vi "Construct.vi"(6 "Bulk Size (1)":i32=1, 7 "Use system decimal point (F)":bool, 8 "error in (no error)":errorcluster, 9 "Constants":cluster{"name":string, "value":dbl}[](array[cluster]), 10 "Expression":string, 11 "muExpr in":refnum<class "mupExpr.lvclass">) -> (0 "error out":errorcluster, 1 "error details":T1, 2 "Variable Names":string[](array[string]), 3 "mupExpr out":refnum<class "mupExpr.lvclass">)   [LabVIEW 2015, in "mupExpr.lvclass"]
doc: "Construct a new muExpr instance. Input an expression or a set of expressions.\nReturns the expression handle and the list of variables found in the expression.\n\nOptionally input a list of constant name-value pairs.\n\nSet \"Use system decimal point\" to true if you want to adapt to the system's decimal point. If the system's decimal point is a comma, the argument separator will be changed to a semi-colon. The default decimal point is a period. The default argument separator is a comma.\n\nSet Bulk Size sets the range for bulk mode evaluations. Default is 1 (single result)."
uses:
  mupExpr.lvclass
  mupExpr.lvclass/mupExpr.ctl
  mupLib/mupLibPath.vi
  mupLib/mupCheckError.vi
  <vilib>/Utility/error.llb/Error Cluster From Error Code.vi
  mupLib/mupLib.lvlib
panel:
  # "Construct a new muExpr instance. Input an expression or a set of expressions.\nReturns the expression handle and the list of variables found in the expression (for convenience)."
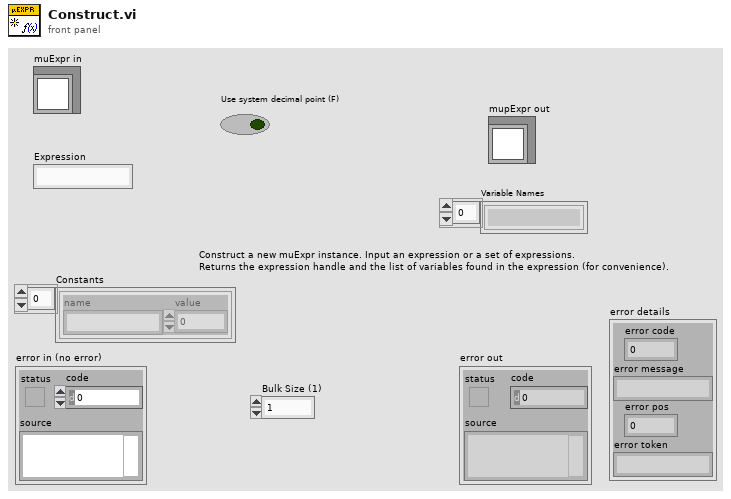
[diagram p1: front panel]
types:
  T1 = cluster{"error code":i32, "error message":string, "error pos":i32, "error token":string}
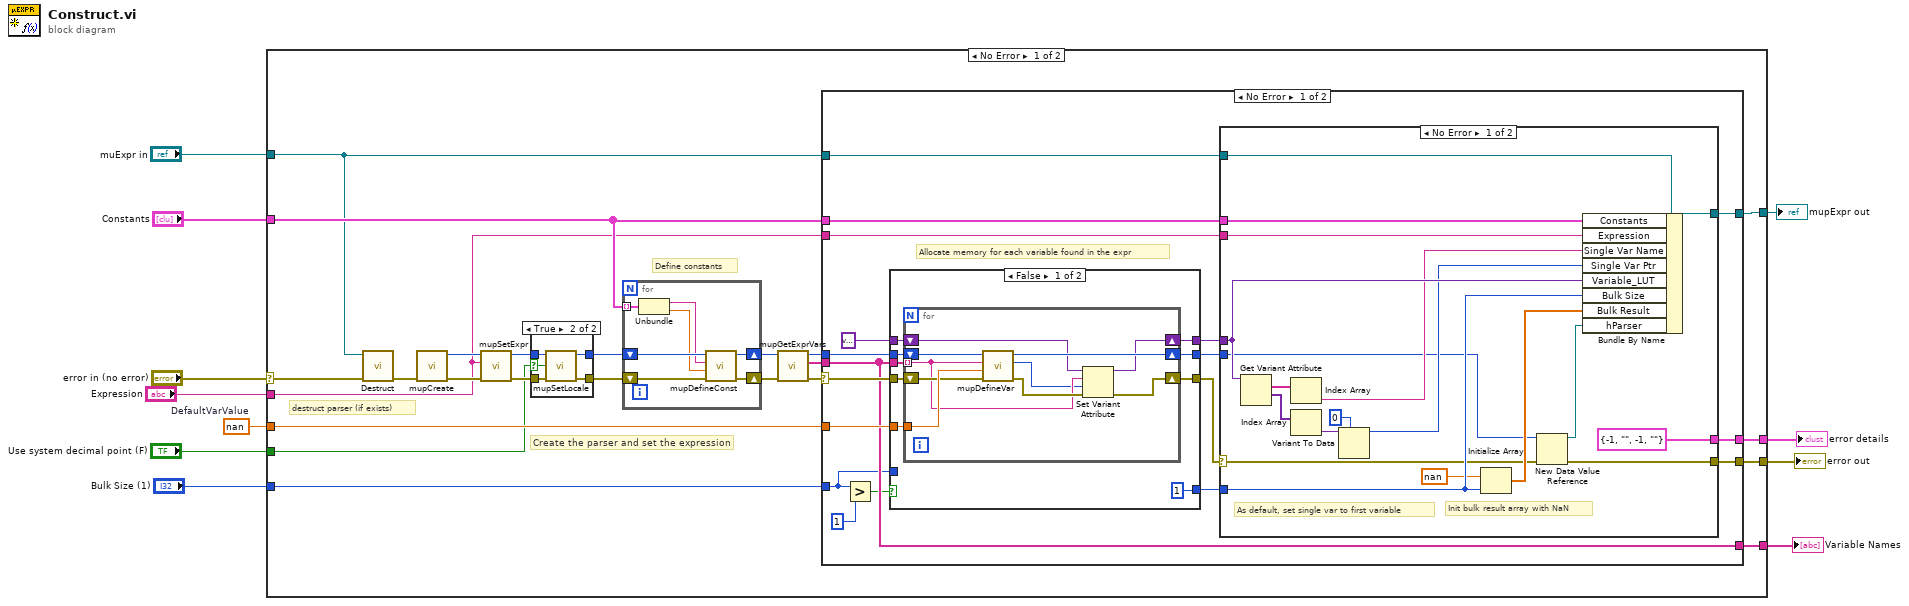
[diagram p0: block diagram]
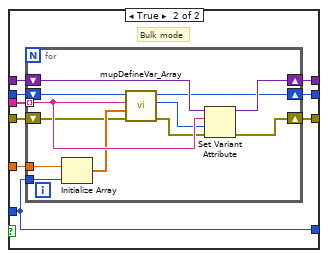
[diagram p3: hidden frame]
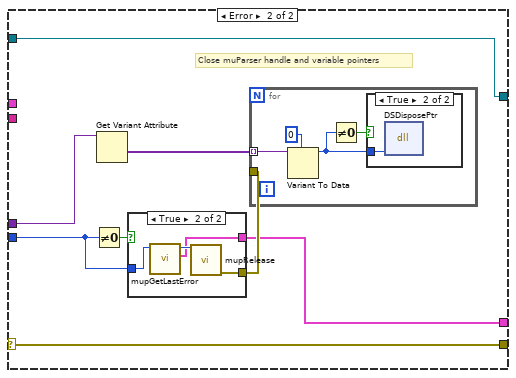
[diagram p4: hidden frame]
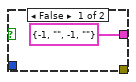
[diagram p5: hidden frame]
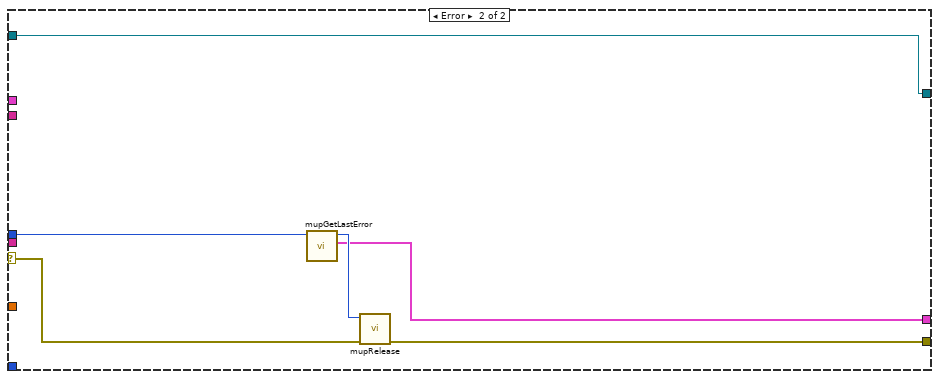
[diagram p7: hidden frame]
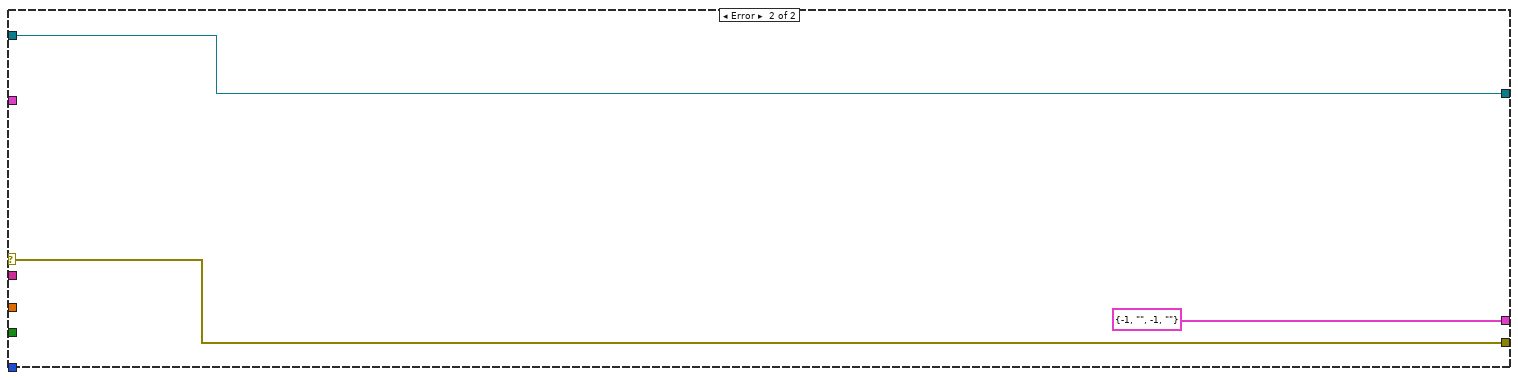
[diagram p8: hidden frame]
diagram:
  w8 = nan  # DefaultVarValue
  n1 = case shown="No Error" "error in (no error)" {
    selector: "error in (no error)" -> [w14 w152]
    tunnel: "Expression" -> [w12 _]
    tunnel: [w34 w150] -> w3
    tunnel: [w33 w152] -> w10
    tunnel: w8 -> [w32 _]
    tunnel: [w31 _] -> w7
    tunnel: "Use system decimal point (F)" -> [w19 _]
    tunnel: "Constants" -> [w17 _]
    tunnel: "Bulk Size (1)" -> [w18 _]
    tunnel: [w16 T1 {"error code"=-1, "error message"="", "error pos"=-1, "error token"=""} ("error details")] -> w2
    tunnel: "muExpr in" -> [w15 w150]
    frame No Error {
      # "destruct parser (if exists)"
      # "Define constants"
      # "Create the parser and set the expression"
      n2 = call-dynamic "Destruct.vi"("error in (no error)"=w14, "muExpr in"=w15) -> ("error out"=w13:errorcluster)  [unwired: 9 in]
      n3 = call "mupCreate.vi"("error in (no error)"=w13) -> ("error out"=w26:errorcluster, "hParser out"=w27:u64)  [unwired: 9 in]
      n4 = call "mupSetExpr.vi"("error in (no error)"=w26, "szExpr"=w12, "muPar in"=w27) -> ("error out"=w25:errorcluster, "muPar out"=w24:u64)  [unwired: 7 in]
      n5 = case shown="True" w19 {
        selector: w19 -> [_ w37]
        tunnel: w25 -> [w35 w41]
        tunnel: w24 -> [w36 w40]
        tunnel: [w36 w39] -> w23
        tunnel: [w35 w38] -> w21
        frame False {
        }
        frame True {
          n6 = call "mupSetLocale.vi"("error in (no error)"=w41, "Use system decimal point (T)"=w37, "hParser in"=w40) -> ("error out"=w38:errorcluster, "hParser out"=w39:u64)  [unwired: 7 in]
        }
      }
      n7 = for {
        shift-right: [w47] -> w22
        shift-left: w23 -> [w48]
        shift-right: [w45] -> w20
        shift-left: w21 -> [w46]
        tunnel: w17 -> [w44] mode=indexing
        n8 = Unbundle(w44) -> ("name"=w43:string, "value"=w42:dbl)
        n9 = call "mupDefineConst.vi"("error in (no error)"=w46, "Value"=w42, "constName"=w43, "hParser in"=w48) -> ("error out"=w45:errorcluster, "hParser out"=w47:u64)  [unwired: 6 in]
      }
      n10 = call "mupGetExprVars.vi"("error in (no error)"=w20, "hParser in"=w22) -> ("error out"=w29:errorcluster, "varNames"=w28:string[], "hParser out"=w30:u64)  [unwired: 5 in, 2 out]
      n11 = case shown="No Error" w29 {
        selector: w29 -> [w61 w146]
        tunnel: [w66 w144] -> w34
        tunnel: [w65 w149] -> w33
        tunnel: w32 -> [w62 _]
        tunnel: w30 -> [w63 w147]
        tunnel: [w57 _] -> w31
        tunnel: w28 -> [w57 _]
        tunnel: w18 -> [w54 _]
        tunnel: w17 -> [w53 _]
        tunnel: [w51 w145] -> w16
        tunnel: w15 -> [w50 w144]
        tunnel: w12 -> [w49 _]
        frame No Error {
          # "Allocate memory for each variable found in the expr"
          n12 = Greater?(x=w54, y=1) -> (0:w55:bool)
          n13 = case shown="False" w55 {
            tunnel: variant -> [w75 w94]
            tunnel: w63 -> [w74 w93]
            tunnel: w62 -> [w73 w92]
            tunnel: w61 -> [w72 w91]
            tunnel: [w71 w90] -> w60
            tunnel: [w70 w89] -> w59
            tunnel: [w69 w88] -> w58
            tunnel: w57 -> [w68 w87]
            tunnel: w54 -> [_ w86]
            tunnel: [1 ("Bulk Size (1)") w86] -> w52
            frame False {
              n14 = for {
                tunnel: w68 -> [w78] mode=indexing
                shift-right: [w79] -> w69
                shift-left: w75 -> [w80]
                shift-right: [w84] -> w70
                shift-left: w74 -> [w85]
                tunnel: w73 -> [w83]
                shift-right: [w76] -> w71
                shift-left: w72 -> [w82]
                n15 = call "mupDefineVar.vi"("error in (no error)"=w82, "initValue"=w83, "varName"=w78, "hParser in"=w85) -> ("error out"=w81:errorcluster, "varAddr"=w77:u64, "hParser out"=w84:u64)  [unwired: 5 in]
                n16 = Set Variant Attribute(Variant=w80, name=w78, value=w77, error in=w81) -> (Variant out=w79:variant, error out=w76:errorcluster)  [unwired: 1 out]
              }
            }
            frame True {
              # "Bulk mode"
              n17 = for {
                tunnel: w87 -> [w99] mode=indexing
                shift-right: [w105] -> w88
                shift-left: w94 -> [w106]
                shift-right: [w100] -> w89
                shift-left: w93 -> [w101]
                tunnel: w92 -> [w103]
                shift-right: [w104] -> w90
                shift-left: w91 -> [w97]
                tunnel: w86 -> [w102]
                n18 = Initialize Array(w103, w102) -> (w98:dbl[])
                n19 = call "mupDefineVar_Array.vi"("error in (no error)"=w97, "initValue"=w98, "varName"=w99, "hParser in"=w101) -> ("error out"=w96:errorcluster, "varAddr"=w95:u64, "hParser out"=w100:u64)  [unwired: 5 in]
                n20 = Set Variant Attribute(Variant=w106, name=w99, value=w95, error in=w96) -> (Variant out=w105:variant, error out=w104:errorcluster)  [unwired: 1 out]
              }
            }
          }
          n21 = case shown="No Error" w60 {
            selector: w60 -> [w107 w129]
            tunnel: [w113 w126] -> w66
            tunnel: w59 -> [w109 w132]
            tunnel: w58 -> [w125 w131]
            tunnel: [w110 w129] -> w65
            tunnel: w53 -> [w118 _]
            tunnel: w52 -> [w117 _]
            tunnel: [T1 {"error code"=-1, "error message"="", "error pos"=-1, "error token"=""} ("error details") w127] -> w51
            tunnel: w50 -> [w112 w126]
            tunnel: w49 -> [w108 _]
            frame No Error {
              # "As default, set single var to first variable"
              # "Init bulk result array with NaN"
              n22 = Get Variant Attribute(Variant=w125) -> (names=w124:string[], values=w123:variant[])  [unwired: 3 in, 2 out]
              n23 = Index Array(array=w124) -> (element=w120:string)  [unwired: 1 in]
              n24 = Index Array(array=w123) -> (element=w122:variant)  [unwired: 1 in]
              n25 = Variant To Data(type=u64 0, Variant=w122) -> (data=w119:u64)  [unwired: 1 in, 1 out]
              n26 = Initialize Array(nan ("element"), w117) -> (w115:dbl[])
              n27 = New Data Value Reference(data value=w109, error in=w107) -> (data value reference=w111:refnum<data-value>, error out=w110:errorcluster)
              n28 = Bundle By Name(cluster=w112, "Constants"=w118, "Expression"=w108, "Single Var Name"=w120, "Single Var Ptr"=w119, "Variable_LUT"=w125, "Bulk Size"=w117, "Bulk Result"=w115, "hParser"=w111) -> (w113:refnum<class "mupExpr.lvclass">)
            }
            frame Error {
              # "Close muParser handle and variable pointers"
              n29 = Not Equal To 0?(x=w132) -> (x != 0?=w133:bool)
              n30 = Get Variant Attribute(Variant=w131) -> (values=w130:variant[])  [unwired: 3 in, 3 out]
              n31 = case shown="True" w133 {
                tunnel: [_ w138] -> w128
                tunnel: w132 -> [_ w137]
                tunnel: [T1 {"error code"=-1, "error message"="", "error pos"=-1, "error token"=""} ("error details") w135] -> w127
                frame False {
                }
                frame True {
                  n32 = call "mupGetLastError.vi"("hParser in"=w137) -> ("error details"=w135:T1, "hParser out"=w136:u64)  [unwired: 8 in, 1 out]
                  n33 = call "mupRelease.vi"("hParser in"=w136) -> ("error out"=w138:errorcluster)  [unwired: 10 in]
                }
              }
              n34 = for {
                tunnel: w130 -> [w142] mode=indexing
                tunnel: w128 -> [_]
                n35 = Variant To Data(type=u64 0, Variant=w142) -> (data=w140:u64)  [unwired: 1 in, 1 out]
                n36 = Not Equal To 0?(x=w140) -> (x != 0?=w139:bool)
                n37 = case shown="True" w139 {
                  tunnel: w140 -> [_ w143]
                  frame False {
                  }
                  frame True {
                    n38 = dll-call lib="LabVIEW" fn="DSDisposePtr"("ptr"=w143) -> ()  [unwired: 5 in, 2 out]
                  }
                }
              }
            }
          }
        }
        frame Error {
          n39 = call "mupGetLastError.vi"("hParser in"=w147) -> ("error details"=w145:T1, "hParser out"=w148:u64)  [unwired: 8 in, 1 out]
          n40 = call "mupRelease.vi"("error in (no error)"=w146, "hParser in"=w148) -> ("error out"=w149:errorcluster)  [unwired: 9 in]
        }
      }
    }
    frame Error {
    }
  }
  "error out" <- w10
  "Variable Names" <- w7
  "mupExpr out" <- w3
  "error details" <- w2
